vi "Get Table Path.vi"(8 "error in (no error)":errorcluster, 10 "Table":string, 11 "Data.PG":refnum<class "Data.PGSQL.lvclass">) -> (0 "error out":errorcluster, 2 "Table Path":string, 3 "Data.PG out":refnum<class "Data.PGSQL.lvclass">)   [LabVIEW 2013, in "Data.PGSQL.lvclass"]
uses:
  Data.PGSQL.lvclass
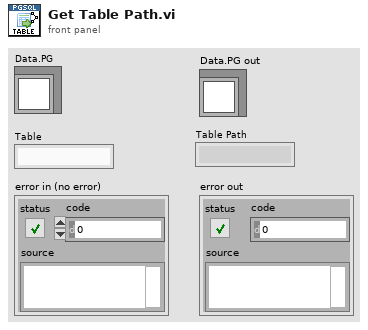
[diagram p1: front panel]
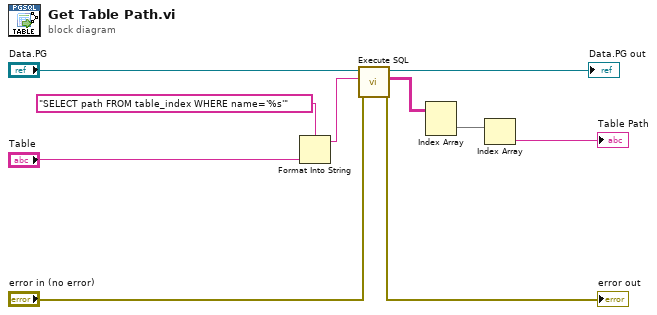
[diagram p0: block diagram]
diagram:
  n1 = Format Into String(format string="SELECT path FROM table_index WHERE name='%s'", "Table") -> (resulting string=w7:string)  [unwired: 2 in, 1 out]
  n2 = call "Execute SQL.vi"("error in"="error in (no error)", "SQL"=w7, "Data.PG"="Data.PG") -> ("error out"=→"error out":errorcluster, "Result"=w2:string[][], "Data.PG out"=→"Data.PG out":refnum<class "Data.PGSQL.lvclass">)  [unwired: 6 in]
  n3 = Index Array(array=w2) -> (element=w9:string[])  [unwired: 2 in]
  n4 = Index Array(array=w9) -> (element=→"Table Path":string)  [unwired: 1 in]
